vi "wire to tag bus.vi"(7 "unique key":string, 8 "error in":errorcluster, 10 "wire data":string, 11 "data table in":T1) -> (0 "error out":errorcluster, 3 "data table out":T1)   [LabVIEW 2013, in "TEC runtime.lvclass"]
uses:
  TEC runtime.lvclass
  <vilib>/NI/Tag Bus/table/data table.ctl
  <vilib>/NI/Tag Bus/table/data table.lvlib
  <vilib>/NI/Configuration Framework/NISE_CEF_TreeControl.lvlib
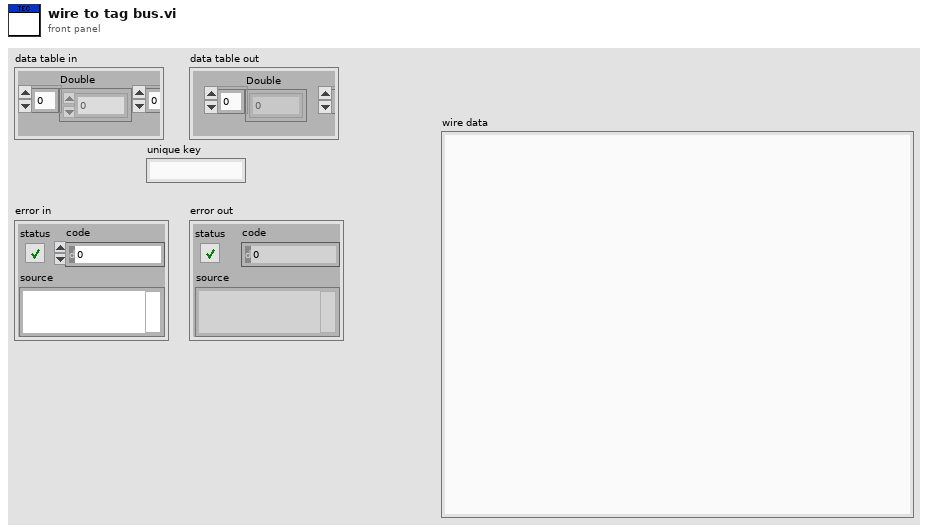
[diagram p1: front panel]
types:
  T1 = typedef "tag bus.lvlib/data table.lvlib/data table.ctl" = cluster{"Double":dbl[], "Single":sgl[], "I64":i64[], "I32":i32[], "I16":i16[], "I8":i8[], "U64":u64[], "U32":u32[], "U16":u16[], "U8":u8[], "Boolean":bool[], "String":string[], "Array of Double":cluster{"DBL Array":dbl[]}[], "Array of Single":cluster{"SGL Array":sgl[]}[], "Array of I64":cluster{"I64 Array":i64[]}[], "Array of I32":cluster{"I32 Array":i32[]}[], "Array of I16":cluster{"I16 Array":i16[]}[], "Array of I8":cluster{"I8 Array":i8[]}[], "Array of U64":cluster{"U64 Array":u64[]}[], "Array of U32":cluster{"U32 Array":u32[]}[], "Array of U16":cluster{"U16 Array":u16[]}[], "Array of U8":cluster{"U8 Array":u8[]}[], "Array of Boolean":cluster{"Boolean Array":bool[]}[], "Array of String":cluster{"String Array":string[]}[]}
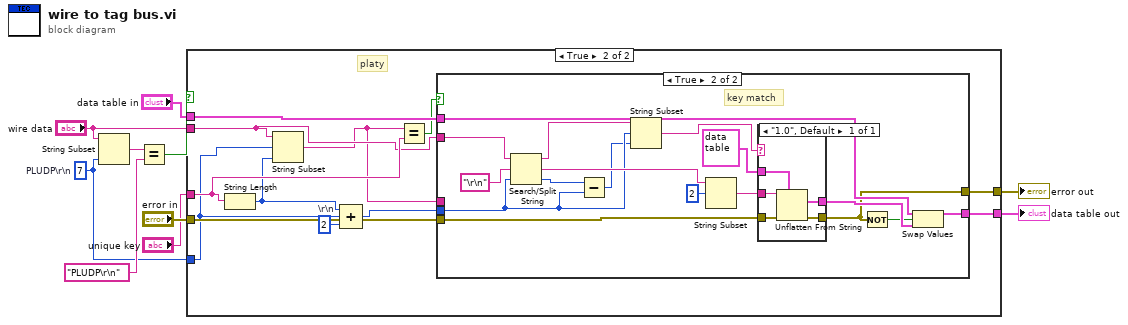
[diagram p0: block diagram]
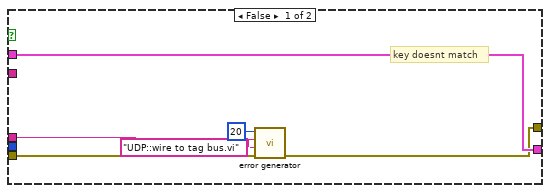
[diagram p3: hidden frame]
diagram:
  w1 = 7  # PLUDP\r\n
  n1 = String Subset(string="wire data", length (rest)=w1) -> (substring=w5:string)  [unwired: 1 in]
  n2 = Equal?(x=w5, y="PLUDP\r\n" ("string")) -> (x = y?=w3:bool)
  n3 = case shown="True" w3 {
    tunnel: "error in" -> [w11 w24]
    tunnel: "data table in" -> [w12 w23]
    tunnel: [w12 w22] -> w8
    tunnel: [w11 w21] -> w7
    tunnel: "wire data" -> [_ w18]
    tunnel: "unique key" -> [_ w19]
    tunnel: w1 -> [_ w16]
    frame False {
      # "not platy, ignore"
    }
    frame True {
      w15 = 2  # \r\n
      # "platy"
      n4 = String Length(string=w19) -> (length=w17:i32)
      n5 = String Subset(string=w18, offset (0)=w16, length (rest)=w17) -> (substring=w13:string)
      n6 = Compound Arithmetic op=ADD(w17, w16, w15) -> (w14:i32)
      n7 = Equal?(x=w13, y=w19) -> (x = y?=w20:bool)
      n8 = case shown="True" w20 {
        tunnel: w24 -> [w29 w47]
        tunnel: w23 -> [w30 w45]
        tunnel: [w30 w44] -> w22
        tunnel: [w28 w43] -> w21
        tunnel: w18 -> [_ w38]
        tunnel: w14 -> [_ w35]
        tunnel: w13 -> [w26 _]
        frame False {
          # "key doesnt match"
          n9 = call <vilib>:"error generator.vi"("error in"=w29, "source"="UDP::wire to tag bus.vi", "append error message"=w26, "error code (0)"=20) -> ("error out"=w28:errorcluster)  [unwired: 5 in]
        }
        frame True {
          # "key match"
          n10 = Search/Split String(string=w38, search string/char (-)="\r\n" ("string"), offset (0)=w35) -> (substring before match=w32:string, match + rest of string=w40:string, offset of match=w34:i32)
          n11 = Subtract(x=w34, y=w35) -> (x-y=w33:i32)
          n12 = String Subset(string=w32, offset (0)=w35, length (rest)=w33) -> (substring=w31:string)
          n13 = String Subset(string=w40, offset (0)=2) -> (substring=w39:string)  [unwired: 1 in]
          n14 = case shown="\"1.0\", Default" w31 {
            tunnel: w39 -> [w49]
            tunnel: w47 -> [w52]
            tunnel: [w48] -> w46
            tunnel: [w51] -> w43
            tunnel: T1 {"Double"=[], "Single"=[], "I64"=[], "I32"=[], "I16"=[], "I8"=[], "U64"=[], "U32"=[], "U16"=[], "U8"=[], "Boolean"=[], "String"=[], "Array of Double"=[], "Array of Single"=[], "Array of I64"=[], "Array of I32"=[], "Array of I16"=[], "Array of I8"=[], "Array of U64"=[], "Array of U32"=[], "Array of U16"=[], "Array of U8"=[], "Array of Boolean"=[], "Array of String"=[]} ("data table in") -> [w50]
            frame "1.0", Default {
              n15 = Unflatten From String(type=w50, binary string=w49, error in (no error)=w52) -> (value=w48:T1, error out=w51:errorcluster)  [unwired: 2 in, 1 out]
            }
          }
          n16 = Not(x=w43) -> (.not. x?=w42:bool)
          n17 = Swap Values(12:w45, 13:w42, 14:w46) -> (1:w44:T1)  [unwired: 1 out]
        }
      }
    }
  }
  "error out" <- w7
  "data table out" <- w8
